vi "Autunomous_Initilization.vi"() -> (0 "errror out":errorcluster)   [LabVIEW 2018]
uses:
  Global_Variables/Refnum_Names.vi
  <vilib>/Rock Robotics/WPI/Utilities/WPI_GetSetVariantRefNum.vi
  Global_Variables/Drive_Globals.vi
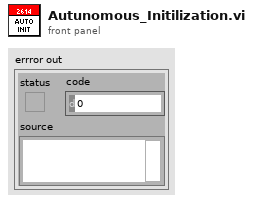
[diagram p1: front panel]
types:
  T1 = typedef "CTRE_PigeonIMU_DeviceRef.ctl" = cluster{"DeviceStatus":errorcluster, "Device Number":u8, "Type":T2, "Device ID":u32, "Handle":u64, "UsageFrame":u32, "Library Path":path}
  T2 = typedef "CTRE_PigeonIMU_ConnectionType.ctl" = u32
  T3 = typedef "WPI_CompressorDevRef.ctl" = cluster{"DevStatus":errorcluster, "Pneumatics Control Module":u8}
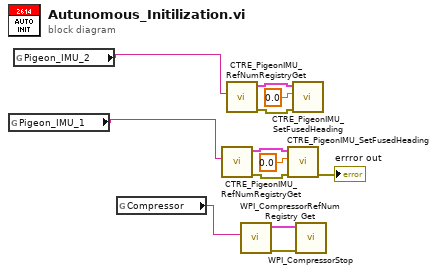
[diagram p0: block diagram]
diagram:
  n1 = global read "Drive_Globals.vi" "Pigeon_IMU_1"() -> (w5:string)
  n2 = global read "Drive_Globals.vi" "Pigeon_IMU_2"() -> (w4:string)
  n3 = global read "Refnum_Names.vi" "Compressor"() -> (w6:string)
  n4 = call <vilib>:"CTRE_PigeonIMU_RefNumRegistryGet.vi"("refnum name"=w5) -> ("error out"=w10:errorcluster, "PigeonIMUDevRef"=w11:T1)  [unwired: 9 in]
  n5 = call <vilib>:"CTRE_PigeonIMU_RefNumRegistryGet.vi"("refnum name"=w4) -> ("error out"=w3:errorcluster, "PigeonIMUDevRef"=w2:T1)  [unwired: 9 in]
  n6 = call <vilib>:"WPI_CompressorRefNum Registry Get.vi"("refnum name"=w6) -> ("error out"=w7:errorcluster, "CompressorDevRef"=w8:T3)  [unwired: 9 in]
  n7 = call <vilib>:"CTRE_PigeonIMU_SetFusedHeading.vi"("error in (no error)"=w10, "Value"=0.0, "PigeonIMUDevRef 2"=w11) -> ("error out"=→"errror out":errorcluster)  [unwired: 7 in, 1 out]
  n8 = call <vilib>:"CTRE_PigeonIMU_SetFusedHeading.vi"("error in (no error)"=w3, "Value"=0.0, "PigeonIMUDevRef 2"=w2) -> ()  [unwired: 7 in, 2 out]
  n9 = call <vilib>:"WPI_CompressorStop.vi"("error in (no error)"=w7, "CompressorDevRef"=w8) -> ()  [unwired: 8 in, 2 out]
